vi "calibrate.vi"(4 "errorIn":errorcluster, 5 "reverseStepSize":i32, 6 "forwardStepSize":i32, 7 "axis":i32, 8 "referenceIn":refnum<k24>) -> (0 "errorOut":errorcluster, 1 "nForwardSteps":i32, 2 "nReverseSteps":i32, 3 "referenceOut":refnum<k24>)   [LabVIEW 2013]
uses:
  C:/Program Files/Newport/Piezo Motion Control/Newport AG-UC2-UC8 Applet/Samples/LabVIEW 2009/AgilisCmdLib.dll
  Program Files/Newport/Piezo Motion Control/Newport AG-UC2-UC8 Applet/Samples/LabVIEW 2009/AgilisCmdLib.dll
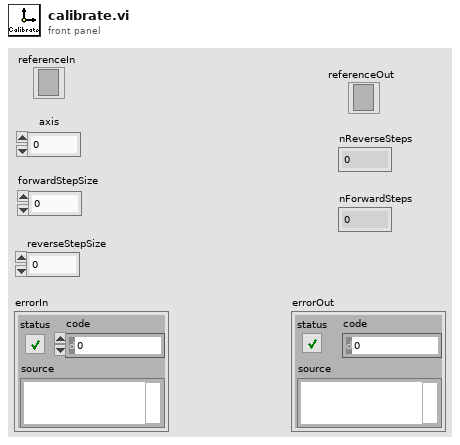
[diagram p1: front panel]
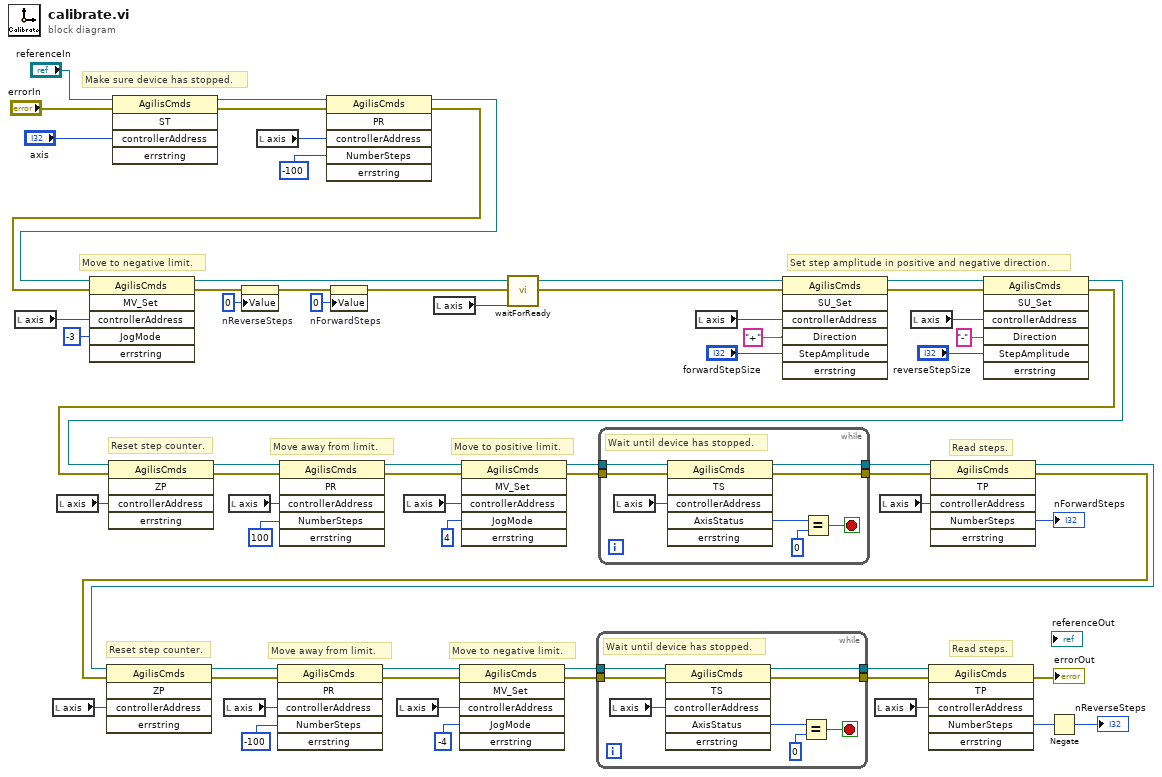
[diagram p0: block diagram]
diagram:
  # "Make sure device has stopped."
  # "Read steps."
  # "Read steps."
  # "Move to negative limit."
  # "Move away from limit."
  # "Reset step counter."
  # "Move to positive limit."
  # "Move away from limit."
  # "Reset step counter."
  # "Set step amplitude in positive and negative direction."
  # "Move to negative limit."
  n1 = local read "axis"() -> (w12:i32)
  n2 = local read "axis"() -> (w26:i32)
  n3 = local read "axis"() -> (w53:i32)
  n4 = invoke class="AgilisCmds" method="ST"(reference="referenceIn", error in="errorIn", "controllerAddress"="axis") -> (reference out=w10:refnum<k24>, error out=w8:errorcluster)  [unwired: 2 in, 3 out]
  n5 = local read "axis"() -> (w25:i32)
  n6 = local read "axis"() -> (w50:i32)
  n7 = local read "axis"() -> (w9:i32)
  n8 = invoke class="AgilisCmds" method="PR"(reference=w10, error in=w8, "controllerAddress"=w9, "NumberSteps"=i64 -100) -> (reference out=w7:refnum<k24>, error out=w6:errorcluster)  [unwired: 2 in, 4 out]
  n9 = invoke class="AgilisCmds" method="MV_Set"(reference=w7, error in=w6, "controllerAddress"=w12, "JogMode"=-3) -> (reference out=w5:refnum<k24>, error out=w63:errorcluster)  [unwired: 2 in, 4 out]
  n10 = property on="nReverseSteps" class="DigNum (strict)"(error in=w63, "Value"=0 ("nReverseSteps")) -> (error out=w61:errorcluster)  [unwired: 1 in, 1 out]
  n11 = property on="nForwardSteps" class="DigNum (strict)"(error in=w61, "Value"=0 ("nForwardSteps")) -> (error out=w4:errorcluster)  [unwired: 1 in, 1 out]
  n12 = local read "axis"() -> (w24:i32)
  n13 = local read "axis"() -> (w48:i32)
  n14 = local read "axis"() -> (w3:i32)
  n15 = call "waitForReady.vi"("axis"=w3, "errorIn"=w4, "referenceIn"=w5) -> ("errorOut"=w1:errorcluster, "referenceOut"=w2:refnum<k24>)
  n16 = local read "axis"() -> (w58:i32)
  n17 = invoke class="AgilisCmds" method="SU_Set"(reference=w2, error in=w1, "controllerAddress"=w58, "Direction"="+", "StepAmplitude"="forwardStepSize") -> (reference out=w55:refnum<k24>, error out=w22:errorcluster)  [unwired: 2 in, 5 out]
  n18 = local read "axis"() -> (w23:i32)
  n19 = local read "axis"() -> (w40:i32)
  n20 = local read "axis"() -> (w56:i32)
  n21 = invoke class="AgilisCmds" method="SU_Set"(reference=w55, error in=w22, "controllerAddress"=w56, "Direction"="-", "StepAmplitude"="reverseStepSize") -> (reference out=w17:refnum<k24>, error out=w18:errorcluster)  [unwired: 2 in, 5 out]
  n22 = invoke class="AgilisCmds" method="ZP"(reference=w17, error in=w18, "controllerAddress"=w53) -> (reference out=w52:refnum<k24>, error out=w51:errorcluster)  [unwired: 2 in, 3 out]
  n23 = invoke class="AgilisCmds" method="PR"(reference=w52, error in=w51, "controllerAddress"=w50, "NumberSteps"=i64 100) -> (reference out=w45:refnum<k24>, error out=w46:errorcluster)  [unwired: 2 in, 4 out]
  n24 = invoke class="AgilisCmds" method="MV_Set"(reference=w45, error in=w46, "controllerAddress"=w48, "JogMode"=4) -> (reference out=w44:refnum<k24>, error out=w43:errorcluster)  [unwired: 2 in, 4 out]
  n25 = while {
    tunnel: w43 -> [w69]
    tunnel: w44 -> [w68]
    tunnel: [w67] -> w42
    tunnel: [w66] -> w41
    stop <- w70 stop-if-true
    # "Wait until device has stopped."
    n26 = local read "axis"() -> (w65:i32)
    n27 = invoke class="AgilisCmds" method="TS"(reference=w68, error in=w69, "controllerAddress"=w65) -> (reference out=w67:refnum<k24>, error out=w66:errorcluster, "AxisStatus"=w72:i32)  [unwired: 3 in, 3 out]
    n28 = Equal?(x=w72, y=0) -> (x = y?=w70:bool)
  }
  n29 = invoke class="AgilisCmds" method="TP"(reference=w42, error in=w41, "controllerAddress"=w40) -> (reference out=w27:refnum<k24>, error out=w28:errorcluster, "NumberSteps"=→"nForwardSteps":i32)  [unwired: 3 in, 3 out]
  n30 = invoke class="AgilisCmds" method="ZP"(reference=w27, error in=w28, "controllerAddress"=w26) -> (reference out=w38:refnum<k24>, error out=w37:errorcluster)  [unwired: 2 in, 3 out]
  n31 = invoke class="AgilisCmds" method="PR"(reference=w38, error in=w37, "controllerAddress"=w25, "NumberSteps"=i64 -100) -> (reference out=w33:refnum<k24>, error out=w34:errorcluster)  [unwired: 2 in, 4 out]
  n32 = invoke class="AgilisCmds" method="MV_Set"(reference=w33, error in=w34, "controllerAddress"=w24, "JogMode"=-4) -> (reference out=w32:refnum<k24>, error out=w31:errorcluster)  [unwired: 2 in, 4 out]
  n33 = while {
    tunnel: w31 -> [w77]
    tunnel: w32 -> [w76]
    tunnel: [w75] -> w30
    tunnel: [w74] -> w29
    stop <- w78 stop-if-true
    # "Wait until device has stopped."
    n34 = local read "axis"() -> (w73:i32)
    n35 = invoke class="AgilisCmds" method="TS"(reference=w76, error in=w77, "controllerAddress"=w73) -> (reference out=w75:refnum<k24>, error out=w74:errorcluster, "AxisStatus"=w80:i32)  [unwired: 3 in, 3 out]
    n36 = Equal?(x=w80, y=0) -> (x = y?=w78:bool)
  }
  n37 = invoke class="AgilisCmds" method="TP"(reference=w30, error in=w29, "controllerAddress"=w23) -> (error out=→"errorOut":errorcluster, "NumberSteps"=w20:i32)  [unwired: 3 in, 4 out]
  n38 = Negate(x=w20) -> (-x=→"nReverseSteps":i32)
